vi "Set Clapper Province.vi"(8 "error in":errorcluster, 10 "Enum":T2=enum."Bin Closed", 11 "Auto Notifiers In":T1) -> (0 "error out":errorcluster, 3 "Auto Notifiers Out":T1)   [LabVIEW 2014]
doc: "This Vi will set the Clapper state in the periodic tasks loop then wait until the PID controller has settled then finish execution"
uses:
  Main/Arms/Arm clapper state.ctl
  Auto Notifiers.ctl
  Main/Arms/Arm State.ctl
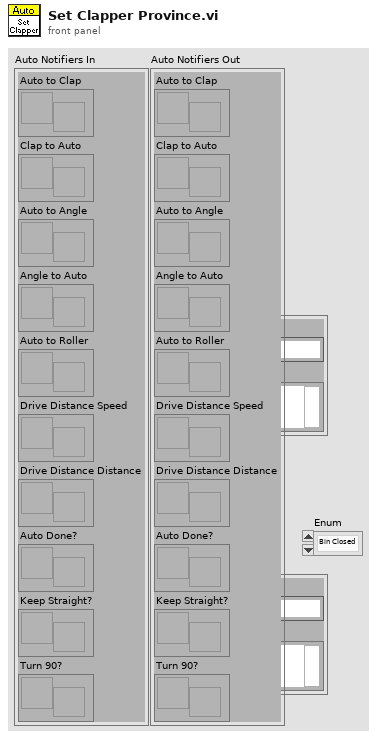
[diagram p1: front panel]
types:
  T1 = typedef "Auto Notifiers.ctl" = cluster{"Auto to Clap":refnum<notifier>, "Clap to Auto":refnum<notifier>, "Auto to Angle":refnum<notifier>, "Angle to Auto":refnum<notifier>, "Auto to Roller":refnum<notifier>, "Drive Distance Speed":refnum<notifier>, "Drive Distance Distance":refnum<notifier>, "Auto Done?":refnum<notifier>, "Keep Straight?":refnum<notifier>, "Turn 90?":refnum<notifier>}
  T2 = typedef "Arm clapper state.ctl" = enum16{"In", "Tote Closed", "Bin Closed", "Straight", "Open"}
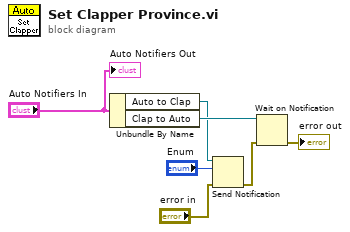
[diagram p0: block diagram]
diagram:
  n1 = Unbundle By Name("Auto Notifiers In") -> ("Auto to Clap"=w2:refnum<notifier>, "Clap to Auto"=w3:refnum<notifier>)
  n2 = Send Notification(notification="Enum", notifier=w2, error in (no error)="error in") -> (error out=w4:errorcluster)  [unwired: 1 out]
  n3 = Wait on Notification(notifier=w3, error in (no error)=w4) -> (error out=→"error out":errorcluster)  [unwired: 2 in, 3 out]
  "Auto Notifiers Out" <- "Auto Notifiers In"
